vi "_Raise Basic Authentication Requested.vi"(4 "WebView2.lvlib:WebView2 Control.lvclass":refnum<class "WebView2 Control.lvclass">, 5 "Event Data":cluster{"sender":refnum<k24>, "e":refnum<k24>}, 6 "Control Ref":refnum<k24>, 7 "Event Common Data":T1) -> ()   [LabVIEW 2025, in "WebView2.lvlib" / "WebView2 Control.lvclass"]
uses:
  WebView2 Control.lvclass
  WebView2 Control.lvclass/WebView2 Control.ctl
  E:/Labview/LV 2023/PPL/PPL Builder/Libs/LV-WebView2/Source/Libs/Microsoft.Web.WebView2.Core.dll
  Libs/Microsoft.Web.WebView2.Core.dll
  Basic Auth Event Data.ctl
  WebView2 Event Filter Interface/WebView2 Event Filter Interface.lvclass
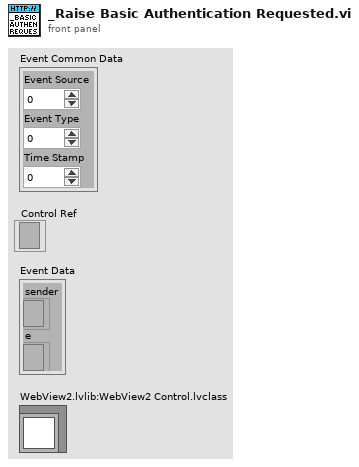
[diagram p1: front panel]
types:
  T1 = cluster{"Event Source":i32, "Event Type":u32, "Time Stamp":u32}
  T2 = typedef "WebView2.lvlib/WebView2 Control.lvclass/Basic Auth Event Data.ctl" = cluster{"Challenge":string, "Uri":string, "Response":refnum<k24>}
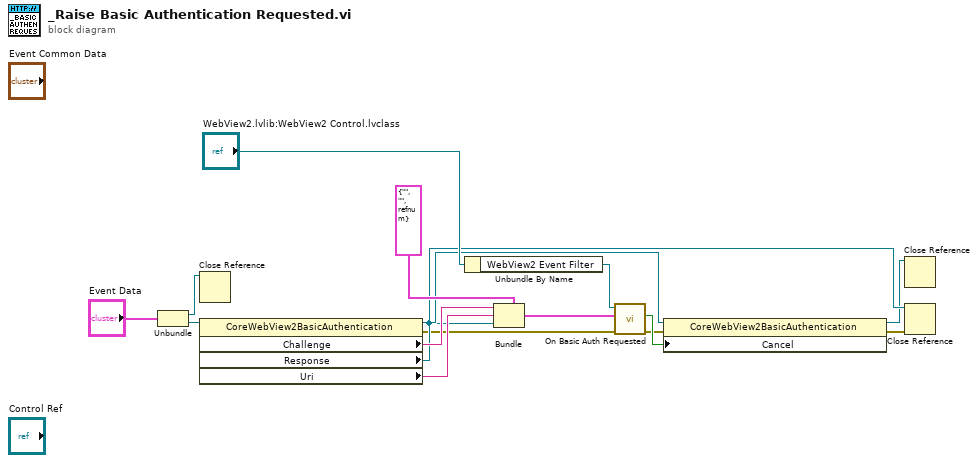
[diagram p0: block diagram]
diagram:
  n1 = Unbundle("Event Data") -> ("sender"=w14:refnum<k24>, "e"=w15:refnum<k24>)
  n2 = Close Reference(reference=w14) -> ()  [unwired: 1 in, 1 out]
  n3 = property class="CoreWebView2BasicAuthentication"(reference=w15) -> (reference out=w7:refnum<k24>, error out=w2:errorcluster, "Challenge"=w13:string, "Response"=w4:refnum<k24>, "Uri"=w12:string)  [unwired: 1 in]
  n4 = Unbundle By Name("WebView2.lvlib:WebView2 Control.lvclass") -> ("WebView2 Event Filter"=w9:refnum<class "WebView2 Event Filter Interface.lvclass">)
  n5 = Bundle(cluster=T2 {"Challenge"="", "Uri"="", "Response"=refnum}, "Challenge"=w13, "Uri"=w12, "Response"=w4) -> (w8:T2)
  n6 = call-dynamic "On Basic Auth Requested.vi"("error in (no error)"=w2, "Data"=w8, "WebView2 Event Filter Interface in"=w9) -> ("error out"=w3:errorcluster, "Cancel"=w6:bool)  [unwired: 7 in]
  n7 = property class="CoreWebView2BasicAuthentication"(reference=w7, error in=w3, "Cancel"=w6) -> (reference out=w1:refnum<k24>, error out=w5:errorcluster)
  n8 = Close Reference(reference=w1) -> ()  [unwired: 1 in, 1 out]
  n9 = Close Reference(reference=w4, error in (no error)=w5) -> ()  [unwired: 1 out]
